vi "240124_Nikon-State.vi"(8 "error in (no error)":errorcluster, 9 "Cluster commandes":T3={"Dia lamp"=TRUE, "Dia lamp intensity"=1689.1304347826087, "Objective"=2, "Light path"=2, "Z pos (µm)"=335593} {"Z pos (µm)" min=0 max=990000 step=100 scale=0.0..990000.0; "Light path" items=["1- Eyepiece"=1, "2- Right"=2, "3- Left + Eyepiece"=3, "4- Left"=4]; "Objective" items=["1- Target"=1, "2- PLAN APO 100X 1,45 Oil"=2, "3- Empty"=3, "4- Empty"=4, "5- Empty"=5, "6- Empty"=6]; "Dia lamp intensity" scale=0.0..2100.0}, 10 "Nikon cluster in":T1, 11 "Cluster in":refnum<vi>) -> (0 "error out":errorcluster, 2 "Cluster µscope":T2, 3 "Nikon cluster out":T1)   [LabVIEW 2014]
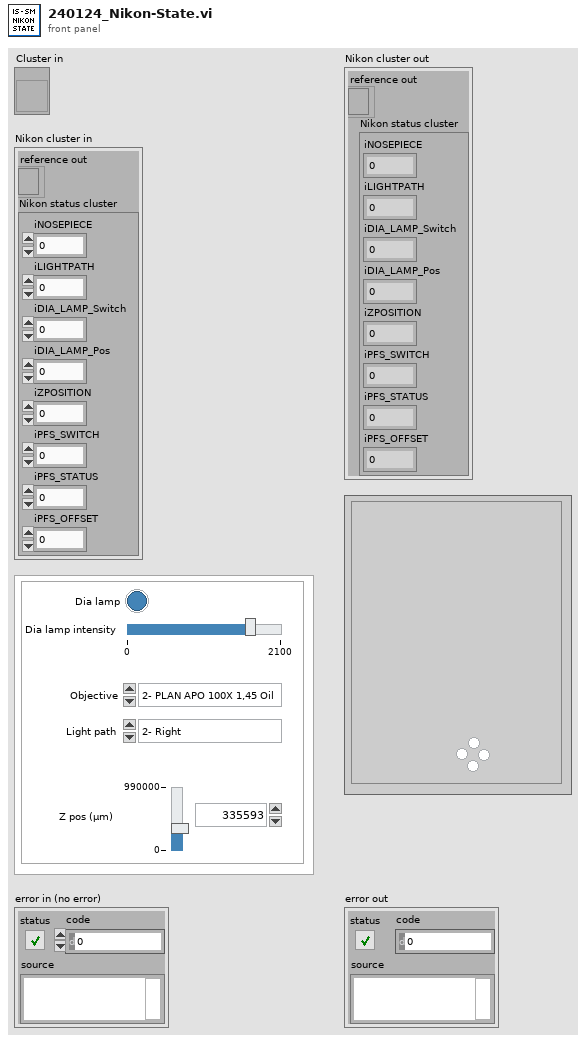
[diagram p1: front panel]
types:
  T1 = cluster{"reference out":refnum<k7>, "Nikon status cluster":cluster{"iNOSEPIECE":i32, "iLIGHTPATH":i32, "iDIA_LAMP_Switch":i32, "iDIA_LAMP_Pos":i32, "iZPOSITION":i32, "iPFS_SWITCH":i32, "iPFS_STATUS":i32, "iPFS_OFFSET":i32}}
  T2 = cluster{"Eyepiece":bool, "Right":bool, "Left + Eyepiece":bool, "Left":bool}
  T3 = cluster{"Dia lamp":bool, "Dia lamp intensity":dbl, "Objective":i32, "Light path":u32, "Z pos (µm)":i32}
  T4 = cluster{"iNOSEPIECE":i32, "iLIGHTPATH":i32, "iDIA_LAMP_Switch":i32, "iDIA_LAMP_Pos":i32, "iZPOSITION":i32, "iPFS_SWITCH":i32, "iPFS_STATUS":i32, "iPFS_OFFSET":i32}
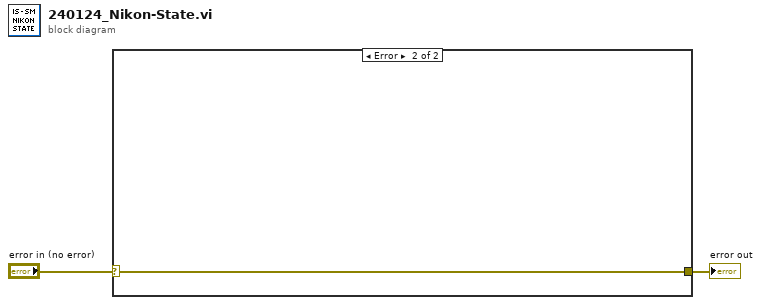
[diagram p0: block diagram]
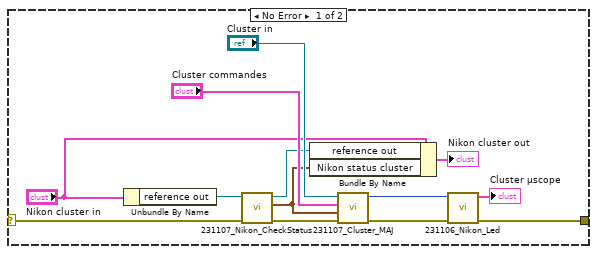
[diagram p2: hidden frame]
diagram:
  n1 = case shown="Error" "error in (no error)" {
    selector: "error in (no error)" -> [w3 w16]
    tunnel: [w15 w16] -> w2
    frame No Error {
      n2 = Unbundle By Name("Nikon cluster in") -> ("reference out"=w4:refnum<k7>)
      n3 = call "231107_Nikon_CheckStatus.vi"("error in"=w3, "NikonTi2AxLib.INikonTi2AxMicroscope"=w4) -> ("error out"=w7:errorcluster, "Nikon status cluster"=w9:T4, "reference out"=w8:refnum<k7>)  [unwired: 7 in]
      n4 = Bundle By Name(cluster="Nikon cluster in", "reference out"=w8, "Nikon status cluster"=w9) -> (→"Nikon cluster out":T1)
      n5 = call "231107_Cluster_MAJ.vi"("error in (no error)"=w7, "Nikon status cluster"=w9, 10:"Cluster commandes"="Cluster commandes", 11:"Cluster commandes"="Cluster in") -> ("error out"=w10:errorcluster, "iLIGHTPATH"=w11:i32)  [unwired: 6 in]
      n6 = call "231106_Nikon_Led.vi"("error in"=w10, "Light path"=w11) -> ("error out"=w15:errorcluster, "Cluster µscope"=→"Cluster µscope":T2)  [unwired: 8 in]
    }
    frame Error {
    }
  }
  "error out" <- w2
